vi "Robotics Environment Simulator.vi"() -> ()   [LabVIEW 2015]
doc: "This VI starts and stops the environment simulator and serves as the master VI for your simulation code. Open and run this VI to display the environment simulator, or open the block diagram to view or modify simulation code."
uses:
  <vilib>/Platform/TimedLoop/XDataNode/timing_clust.ctl
  <vilib>/Platform/TimedLoop/XDataNode/nitl_modes.ctl
  <vilib>/Platform/TimedLoop/XDataNode/wakeup.ctl
  <vilib>/Utility/AngleManip/Degrees to Radians (Scalar DBL).vi
  <vilib>/robotics/Steering/Steering Frame/Apply Steering Frame Velocity to Motors.vi
  LabVIEW Data/MathScriptVIs/MCStatic_35241984432_6b45d99030cf7e9e9617b05270817bf5.vi
  <instcachedir>/0/MCStatic_35241984432_6b45d99030cf7e9e9617b05270817bf5_E3CD1E0DD176482C8238F83966C2E1C4.lvgen/MCStatic_35241984432_6b45d99030cf7e9e9617b05270817bf5_E3CD1E0DD176482C8238F83966C2E1C4_000.vi
  <vilib>/imath/engines/lvmath2/RunTimeEngine/NodeEndStatement/NIMS_NodeEndStatement_Output.vi
  <instcachedir>/0/NIMS_NodeEndStatement_Output_53EC0D466D134D7ABD903AC30B43404B.lvgen/NIMS_NodeEndStatement_Output_53EC0D466D134D7ABD903AC30B43404B_001.vi
  <vilib>/imath/engines/lvmath2/RunTimeEngine/ErrorHandling/NIMS_Finalize Error.vi
  <vilib>/Platform/TimedLoop/XDataNode/XDataNode.xnode
  LabVIEW Data/Coordinates.m
  <vilib>/robotics/Starter Kit/2.0/Sim Host Interface/NI_Robotics_Starter Kit Host_Sim_2.0.lvclass
  <vilib>/robotics/Simulator/NI_Robotics_Simulator.lvlib
  <vilib>/Platform/TimedLoop/XDataNode/XDNodeRunTimeDep.lvlib
  <vilib>/robotics/Steering/Steering Frame/NI_Robotics_Steering Frame.lvclass
  <vilib>/robotics/Starter Kit/Host Interface/NI_Robotics_Starter Kit Host.lvclass
  <vilib>/robotics/Utilities/Scan Angles/NI_Robotics_Scan Angles.lvlib
  <vilib>/robotics/Starter Kit/2.0/NI_Robotics_Starter Kit Host_2.0.lvlib
  <vilib>/Utility/AngleManip/NI_AngleManipulation.lvlib
panel:
  out "angles":dbl[](array[numeric])
  out "distance":dbl[](array[numeric])
  in  "stop":bool
  out "Sensor Data":cluster{"angles (deg)":dbl[], "distances":dbl[]}(graph)
  out "rad_left":dbl
  out "rad_right":dbl
  out "angle_of_goal":dbl
  # "指示左右轮的速度"
  # "整个势场的策略是按照人工势场的方法，适当设定引力和斥力的值\n让小车能够尽量在不碰撞的情况下到达终点，但是考虑到在中途中\n需要应对隔板，所以还加入回退，一旦前方突然检测到障碍物，即\n立刻进入随机走动的回退状态，待转向完毕之后继续前进。"
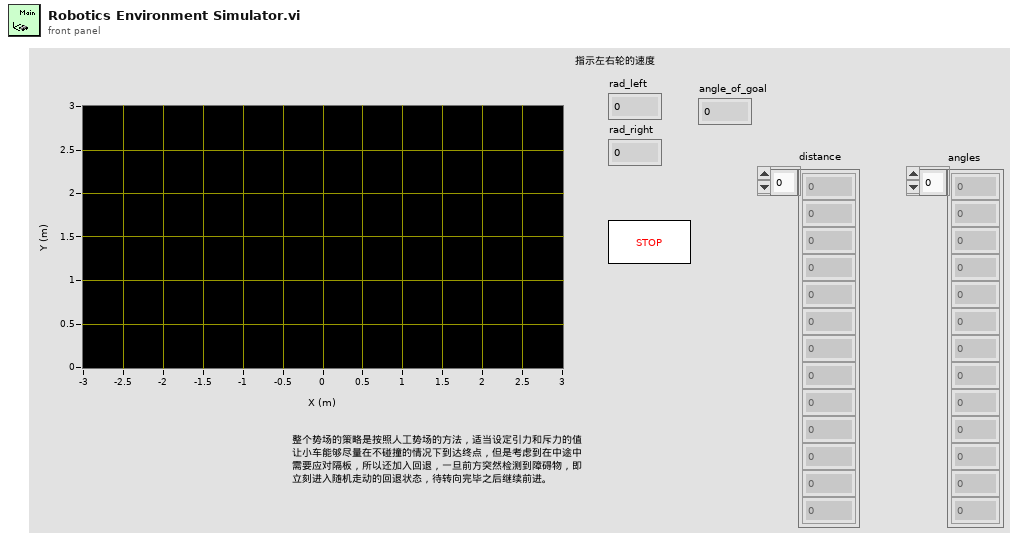
[diagram p1: front panel]
types:
  T1 = typedef "NI_Robotics_Scan Angles.lvlib/Scan Angle Data.ctl" = cluster{"angles":dbl[], "distances":dbl[], "current index":i32, "previous index":i32}
  T2 = typedef "XDNodeRunTimeDep.lvlib/timing_clust.ctl" = cluster{"Expected End [f-1]":u64, "Actual End [f-1]":u64, "Finished Late? [f-1]":bool, "Expected End [i-1]":u64, "Actual End [i-1]":u64, "Finished Late? [i-1]":bool, "Expected Start [i]":u64, "Actual Start [i]":u64, "Expected Start [f]":u64, "Actual Start [f]":u64, "Source Name":string, "Structure Name":string, "Period":i64, "Deadline":i64, "Offset":i64, "Start":i64, "Priority":i32, "Timeout":i32, "Mode":T3, "Wakeup Reason":T4, "Error":errorcluster, "Source Type":string, "Secondary Source Type":string, "Global End Time":u64, "Global Start Time":u64, "Frame Duration":u64, "Iteration Duration":u64, "Assigned CPU":i32, "I/O Scan Engine Mode":u32}
  T3 = typedef "XDNodeRunTimeDep.lvlib/nitl_modes.ctl" = enum32{"No Change", "Process missed periods, maintain original phase", "Discard missed periods, maintain original phase", "Process missed periods, ignore original phase", "Discard missed periods, ignore original phase"}
  T4 = typedef "XDNodeRunTimeDep.lvlib/wakeup.ctl" = enum32{"Normal", "Aborted", "Asynchronous wakeup", "Timing source error", "Timed loop error", "Timeout"}
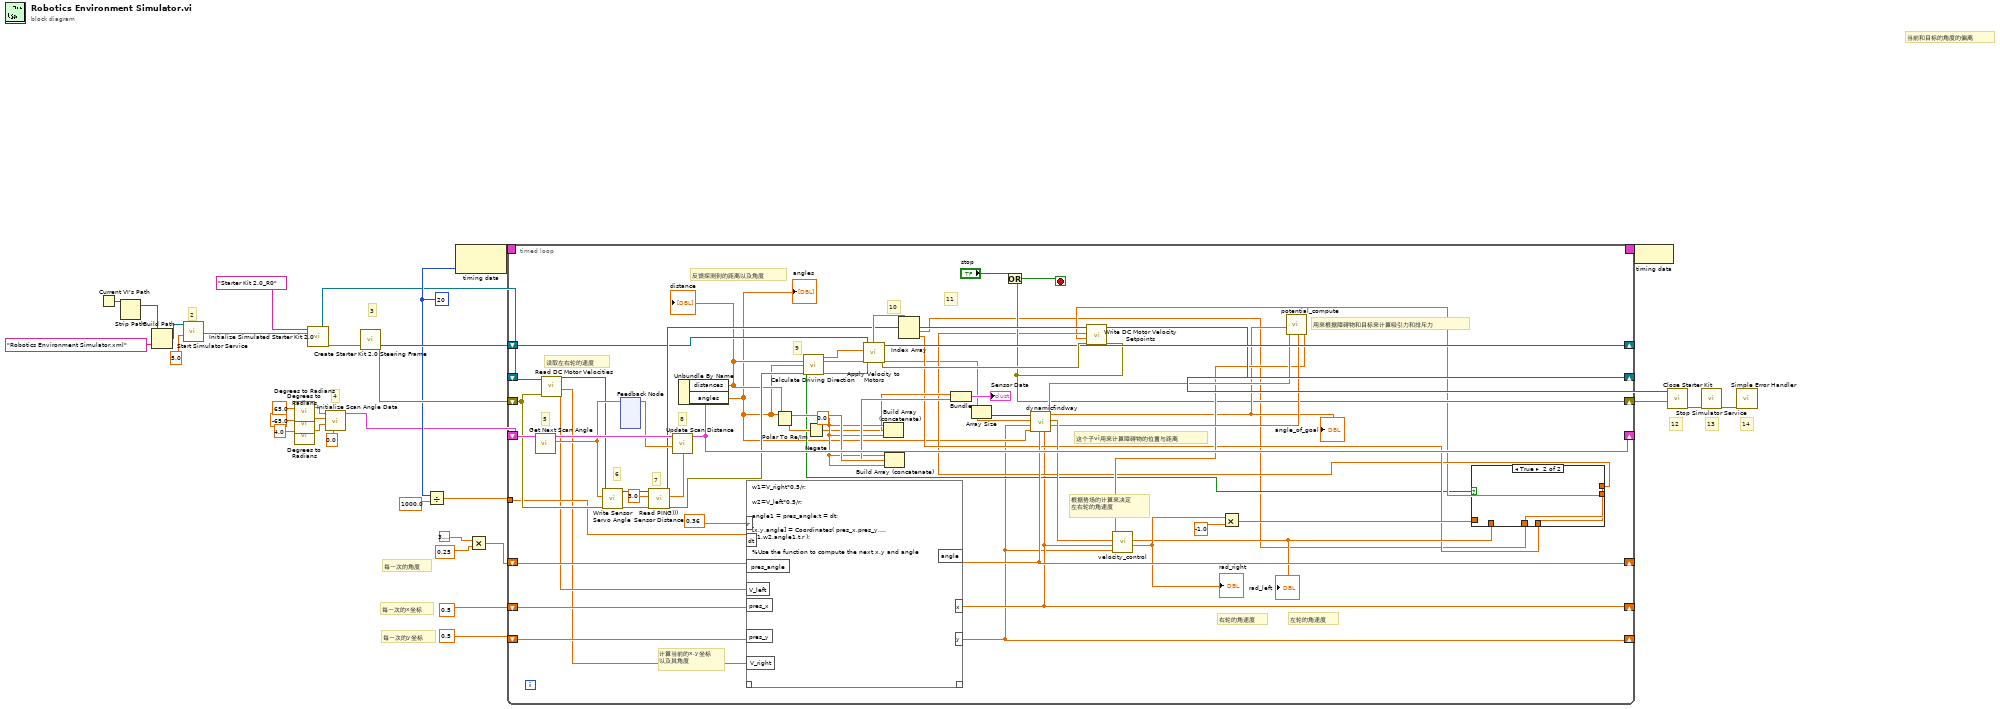
[diagram p0: block diagram]
diagram:
  w13 = i64 20 ("Period")
  # "4"
  # "每一次的y坐标"
  # "每一次的x坐标"
  # "每一次的角度"
  # "当前和目标的角度的偏离"
  # "14"
  # "13"
  # "12"
  # "2"
  # "3"
  n1 = Current VI's Path() -> (path=w32:path)
  n2 = Strip Path(path=w32) -> (stripped path=w31:path)  [unwired: 1 out]
  n3 = Build Path(base path=w31, name or relative path="Robotics Environment Simulator.xml") -> (appended path=w30:path)
  n4 = call <vilib>:"Start Simulator Service.vi"("step size (ms)"=5.0 ("stepsize(ms)"), "manifest file"=w30) -> ("error out"=w14:errorcluster)  [unwired: 9 in]
  n5 = call-poly <vilib>:"Degrees to Radians.vi"("angle (deg)"=65.0 ("max angle")) -> ("angle (rad)"=w11:dbl)  [unwired: 2 in]
  n6 = call-poly <vilib>:"Degrees to Radians.vi"("angle (deg)"=-65.0 ("min angle")) -> ("angle (rad)"=w7:dbl)  [unwired: 2 in]
  n7 = call-poly <vilib>:"Degrees to Radians.vi"("angle (deg)"=4.0 ("scan angle")) -> ("angle (rad)"=w8:dbl)  [unwired: 2 in]
  n8 = call <vilib>:"Initialize Simulated Starter Kit 2.0.vi"("error in (no error)"=w14, "robot ID"="Starter Kit 2.0_R0") -> ("error out"=w25:errorcluster, "simulated starter kit host 2.0 out"=w4:refnum<class "NI_Robotics_Starter Kit Host_Sim_2.0.lvclass">)  [unwired: 8 in]
  n9 = call <vilib>:"Initialize Scan Angle Data.vi"("initial angle (0)"=0.0, "scan angle"=w8, "min angle"=w7, "max angle"=w11) -> ("scan angles"=w5:T1)  [unwired: 6 in, 1 out]
  n10 = call <vilib>:"Create Starter Kit 2.0 Steering Frame.vi"("error in (no error)"=w25) -> ("error out"=w22:errorcluster, "starter kit differential steering frame"=w26:refnum<class "NI_Robotics_Differential Steering Frame.lvclass">)  [unwired: 9 in]
  n11 = Divide(x=w13, y=1000.0) -> (x/y=w15:dbl)
  n12 = node-c288(w13) -> (w28:T2)
  n13 = Multiply(x=3.141592653589793, y=0.25) -> (x*y=w1:dbl)
  n14 = timed-loop {
    shift-right: [w76] -> w24
    shift-left: w4 -> [w63]
    shift-right: [w45] -> w23
    shift-left: w22 -> [w64]
    shift-right: [w78] -> _
    shift-left: w26 -> [w79]
    timing: w28 -> [_]
    timing-out: [_] -> w27
    shift-right: [w75] -> _
    shift-left: w5 -> [w80]
    shift-right: [w55] -> _
    shift-left: w1 -> [w58]
    shift-right: [w35] -> _
    shift-left: 0.5 -> [w59]
    shift-right: [w34] -> _
    shift-left: 0.5 -> [w57]
    tunnel: w15 -> [w56]
    stop <- w77 stop-if-true
    w71 = 0.0 ("element")
    # "反馈探测到的距离以及角度"
    # "读取左右轮的速度"
    # "计算当前的x,y坐标\n以及其角度"
    # "左轮的角速度"
    # "右轮的角速度"
    # "根据势场的计算来决定\n左右轮的角速度"
    # "用来根据障碍物和目标来计算吸引力和排斥力"
    # "这个子vi用来计算障碍物的位置与距离"
    # "7"
    # "6"
    # "11"
    # "10"
    # "9"
    # "8"
    # "5"
    n15 = call <vilib>:"Get Next Scan Angle.vi"("scan angles in"=w80) -> ("new angle"=w87:dbl, "scan angles out"=w90:T1)  [unwired: 9 in]
    n16 = call <vilib>:"Read DC Motor Velocities.vi"("error in (no error)"=w64, "starter kit host in"=w63) -> ("right motor ccw velocity (rad/s)"=w46:dbl, "left motor ccw velocity (rad/s)"=w47:dbl, "starter kit host out"=w62:refnum<class "NI_Robotics_Starter Kit Host_Sim_2.0.lvclass">)  [unwired: 6 in, 1 out]
    n17 = call <vilib>:"Write Sensor Servo Angle.vi"("error in (no error)"=w64, "ccw servo angle (rad)"=w87, "starter kit host in"=w62) -> ("error out"=w84:errorcluster, "starter kit host out"=w85:refnum<class "NI_Robotics_Starter Kit Host_Sim_2.0.lvclass">)  [unwired: 7 in]
    n18 = feedback #1() -> (w89:dbl)  [unwired: 1 in]
    n19 = feedback-in #1(w87) -> ()
    n20 = call <vilib>:"Read PING))) Sensor Distance.vi"("error in (no error)"=w84, "default distance (NaN)"=3.0, "starter kit host in"=w85) -> ("error out"=w66:errorcluster, "distance (m)"=w86:dbl, "starter kit host out"=w83:refnum<class "NI_Robotics_Starter Kit Host_Sim_2.0.lvclass">)  [unwired: 5 in, 1 out]
    n21 = call <vilib>:"Update Scan Distance.vi"("scan angle"=w89, "new scan distance"=w86, "scan angles in"=w90) -> ("scan angles out"=w75:T1)  [unwired: 8 in]
    n22 = Unbundle By Name(w75) -> ("distances"=w37:dbl[], "angles"=w36:dbl[])
    "distance" <- w37
    "angles" <- w36
    n23 = mathscript code="w1=V_right*0.5/r;\n\nw2=V_left*0.5/r;\n\nangle1 = pres_angle;t = dt;\n\n[x,y,angle] = Coordinates( pres_x,pres_y,...\nw1,w2,angle1,t,r );\n\n%Use the function to compute the next x,y and angle"("dt"=w56, "pres_angle"=w58, "V_left"=w47, "V_right"=w46, "pres_x"=w59, "pres_y"=w57, "r"=0.36) -> ("x"=w35:dbl, "angle"=w55:dbl, "y"=w34:dbl)  [unwired: 1 in, 1 out]
    n24 = Polar To Re/Im(2:w36, 3:w37) -> (0:w74:dbl[], 1:w73:dbl[])
    n25 = call "Calculate Driving Direction.vi"("error in (no error)"=w66, "obstacle angles (rad)"=w36, "obstacle distances (m)"=w37) -> ("error out"=w65:errorcluster, "steering frame velocity"=w67:dbl[], "x.or.y?"=w39:bool)  [unwired: 6 in]
    n26 = Negate(x=w74) -> (-x=w69:dbl[])
    n27 = call-poly <vilib>:"Apply Velocity to Motors.vi"("error in (no error)"=w65, "steering frame velocity"=w67, "steering frame in"=w79) -> ("error out"=w82:errorcluster, "ccw motor velocity setpoints"=w88:dbl[], "steering frame out"=w78:refnum<class "NI_Robotics_Differential Steering Frame.lvclass">)  [unwired: 4 in, 2 out]
    n28 = Build Array (concatenate)(w71, w69, w71) -> (w70:dbl[])
    n29 = Build Array (concatenate)(w71, w73, w71) -> (w72:dbl[])
    n30 = Index Array(array=w88) -> (element #1=w38:dbl, element #2=w42:dbl)  [unwired: 2 in]
    n31 = Bundle(w70, w72) -> (→"Sensor Data":cluster{dbl[], dbl[]})  [unwired: 1 in]
    n32 = Array Size(array=w37) -> (size(s)=w48:i32)
    n33 = call "dynamicfindway.vi"("new_x"=w35, "pres_angle"=w55, "angles"=w36, "pres_y"=w34, "distances"=w37, "Numeric"=w48) -> ("angleGoal"=w50:dbl, "distanceGoal"=w53:cdb, "pres_angle"=w54:dbl, "repulsiveForce"=w52:cdb[])  [unwired: 2 in]
    "angle_of_goal" <- w50
    n34 = call "potential_compute.vi"("angle"=w50, "distance"=w53, "repulsiveForce"=w52) -> ("totalForce"=w51:cdb[])  [unwired: 8 in]
    n35 = call "velocity_control.vi"("pres_y"=w34, "pres_x"=w35, "pres_angle"=w54, "totalForce"=w51) -> ("rad_right"=w49:dbl, "rad_left"=w44:dbl)  [unwired: 6 in]
    "rad_right" <- w49
    "rad_left" <- w44
    n36 = Multiply(x=w49, y=-1.0) -> (x*y=w43:dbl)
    n37 = case shown="True" w39 {
      tunnel: w38 -> [_ w95]
      tunnel: w42 -> [_ w94]
      tunnel: [w93 w95] -> w41
      tunnel: [w92 w94] -> w40
      tunnel: w43 -> [w92 _]
      tunnel: w44 -> [w93 _]
      frame False {
        # "r"
        # "l"
      }
      frame True {
      }
    }
    n38 = call <vilib>:"Write DC Motor Velocity Setpoints.vi"("error in (no error)"=w82, "right motor ccw velocity (rad/s)"=w40, "left motor ccw velocity (rad/s)"=w41, "starter kit host in"=w83) -> ("error out"=w45:errorcluster, "starter kit host out"=w76:refnum<class "NI_Robotics_Starter Kit Host_Sim_2.0.lvclass">)  [unwired: 6 in]
    n39 = Or(x=w45, y="stop") -> (x .or. y?=w77:bool)
  }
  n40 = node-c288(w27) -> ()
  n41 = call-dynamic "Close Starter Kit.vi"("error in (no error)"=w23, "starter kit host in"=w24) -> ("error out"=w20:errorcluster)  [unwired: 9 in]
  n42 = call <vilib>:"Stop Simulator Service.vi"("error in (no error)"=w20) -> ("error out"=w19:errorcluster)  [unwired: 10 in]
  n43 = call <vilib>:"Simple Error Handler.vi"("error in (no error)"=w19) -> ()  [unwired: 4 in, 5 out]
